vi "Write Last Switch.vi"(8 "error in (no error)":errorcluster, 10 "Last Switch":timestamp format="%<%H:%M:%S%2u>T", 11 "Output Timer in":refnum<class "Output Timer.lvclass">) -> (0 "error out":errorcluster, 3 "Output Timer out":refnum<class "Output Timer.lvclass">)   [LabVIEW 2013, in "Output Timer.lvclass"]
uses:
  Output Timer.lvclass
  Output Timer.lvclass/Output Timer.ctl
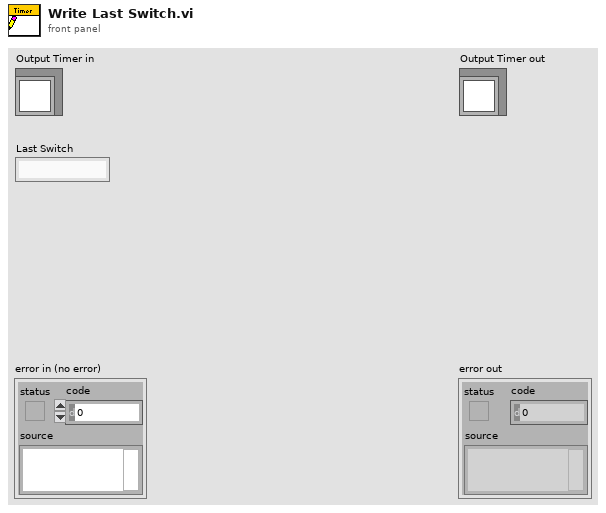
[diagram p1: front panel]
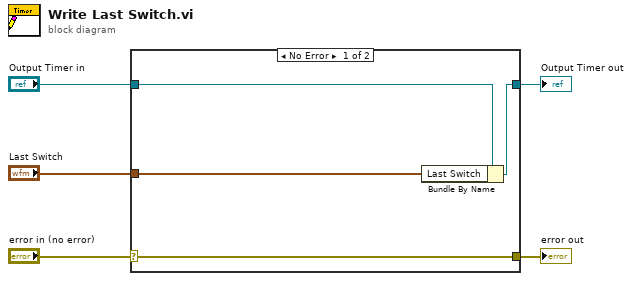
[diagram p0: block diagram]
diagram:
  n1 = case shown="No Error" "error in (no error)" {
    selector: "error in (no error)" -> [w9 w10]
    tunnel: [w9 w10] -> w4
    tunnel: [w7 w11] -> w2
    tunnel: "Output Timer in" -> [w8 w11]
    tunnel: "Last Switch" -> [w6 _]
    frame No Error {
      n2 = Bundle By Name(cluster=w8, "Last Switch"=w6) -> (w7:refnum<class "Output Timer.lvclass">)
    }
    frame Error {
    }
  }
  "error out" <- w4
  "Output Timer out" <- w2
